vi "Read Logo.vi"(8 "error in (no error)":errorcluster, 11 "Instrument Information in":refnum<class "Instrument Information.lvclass">) -> (0 "error out":errorcluster, 2 "Logo2":T1, 3 "Instrument Information out":refnum<class "Instrument Information.lvclass">)   [LabVIEW 2015]
uses:
  Instrument Information.lvclass
  <vilib>/picture/picture.llb/imagedata.ctl
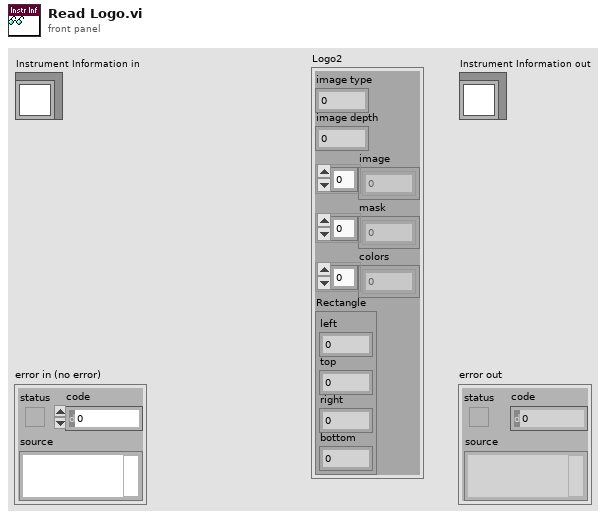
[diagram p1: front panel]
types:
  T1 = typedef "imagedata.ctl" = cluster{"image type":i32, "image depth":i32, "image":u8[], "mask":u8[], "colors":u32[], "Rectangle":cluster{"left":i16, "top":i16, "right":i16, "bottom":i16}}
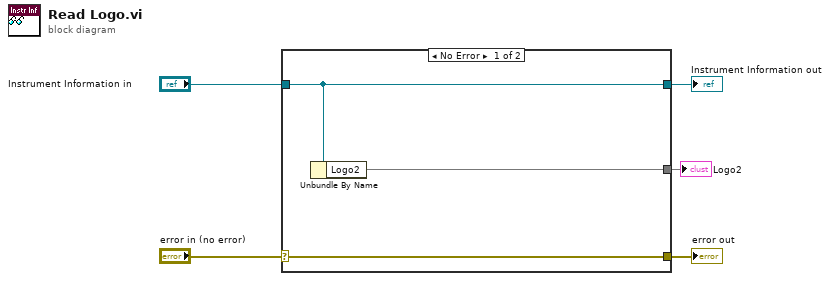
[diagram p0: block diagram]
diagram:
  n1 = case shown="No Error" "error in (no error)" {
    selector: "error in (no error)" -> [w8 w9]
    tunnel: [w8 w9] -> w4
    tunnel: [w7 w10] -> w2
    tunnel: "Instrument Information in" -> [w7 w10]
    tunnel: [w6 _] -> w1
    frame No Error {
      n2 = Unbundle By Name(w7) -> ("Logo2"=w6)
    }
    frame Error {
    }
  }
  "error out" <- w4
  "Instrument Information out" <- w2
  "Logo2" <- w1
